vi "Set Current CCD.vi"(8 "error in (no error)":errorcluster, 11 "CCDCamera in":refnum<class "CCDCamera.lvclass">) -> (0 "error out":errorcluster, 3 "CCDCamera out":refnum<class "CCDCamera.lvclass">)   [LabVIEW 2018, in "CCDCamera.lvclass"]
uses:
  CCDCamera.lvclass
  C:/Users/observer/Desktop/SPARC4_ACS/SPARC4_ACS/Simulated_CCD_Camera/Simulated_CCD_Camera.lvclass
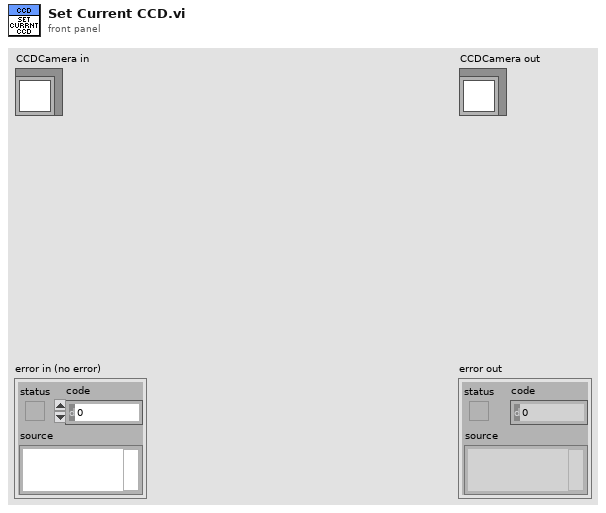
[diagram p1: front panel]
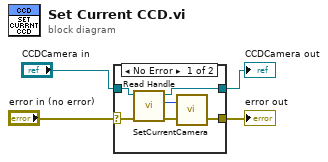
[diagram p0: block diagram]
diagram:
  n1 = case shown="No Error" "error in (no error)" {
    selector: "error in (no error)" -> [w9 w11]
    tunnel: "CCDCamera in" -> [w10 w12]
    tunnel: [w6 w11] -> w2
    tunnel: [w5 w12] -> w1
    frame No Error {
      n2 = call "Read Handle.vi"("error in (no error)"=w9, "Simulated_CCD_Camera in"=w10) -> ("error out"=w7:errorcluster, "Handle"=w8:u16, "Simulated_CCD_Camera out"=w5:refnum<class "CCDCamera.lvclass">)  [unwired: 7 in]
      n3 = call <userlib>:"SetCurrentCamera.vi"("error in (no error)"=w7, "cameraHandle"=w8) -> ("error out"=w6:errorcluster)  [unwired: 1 out]
    }
    frame Error {
    }
  }
  "error out" <- w2
  "CCDCamera out" <- w1
